vi "Subvi AO.vi"(2 "AO channel":refnum<k21>="Connector1/AO0", 10 "Memory label":refnum<k21>="AO0 buffer") -> ()   [LabVIEW 2017]
uses:
  <vilib>/rvi/Emulation/niFpgaGetClockAttributes.vi
  <vilib>/rvi/Emulation/niFpgaSctlEmulationGetInTimedLoop.vi
  <vilib>/rvi/Emulation/niFpgaEmulationReportErrorSimple.vi
  <vilib>/rvi/DataTransferAndStorage/Container/Common/niFpgaContainerExecOnDevCompGetState.vi
  <vilib>/rvi/Emulation/niFpgaEmulationIsFPGAContextNoSignature.vi
  <vilib>/rvi/DataTransferAndStorage/Container/Common/niFpgaContainerGetUniqueNameForEmu.vi
  <vilib>/rvi/Emulation/niFpgaProcessEmulError.vi
  <vilib>/rvi/errors/nirviReportUnexpectedCaseInternalError (U32).vi
  <vilib>/rvi/Memory/Memory_Emulation/niFpgaMemoryEmulationCacheClearOnFirstRun.vi
  <vilib>/rvi/Memory/Memory_Emulation/nirvimemoryEmulationManagerCache_MakeExclusive.vi
  <vilib>/rvi/Memory/Memory_Emulation/niFpgaMemoryEmulationValidateCache.vi
  <vilib>/rvi/Memory/Memory_Emulation/nirvimemoryEmulationManagerCache_InsertValue.vi
  <vilib>/Utility/error.llb/Clear Errors.vi
  <vilib>/rvi/Memory/Memory_Emulation/nirvimemoryEmulationManagerCache_ReleaseExclusive.vi
  <vilib>/rvi/Memory/Memory_Emulation/nirvimemoryEmulationManagerCache_GetValue.vi
  <vilib>/rvi/Memory/Memory_Emulation/nirvimemoryEmulationManagerCache_SetValue.vi
  <vilib>/rvi/Emulation/niFpgaSctlEmulationResourceMgr.vi
  <vilib>/rvi/eio/common/nirviEmuTemplateMethod_errors.vi
  GV trigger.vi
  <vilib>/rvi/Emulation/niFpgaCriticalErrorInLSC.vi
  <vilib>/rvi/DataTransferAndStorage/Container/XNode/niFpgaContainer.xnode
  <vilib>/rvi/Memory/Memory_Emulation/niFpgaMemoryEmulationRefIn.vi
  <vilib>/eio/EIONode/EIONode.xnode
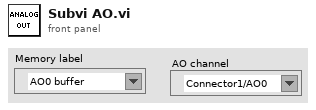
[diagram p1: front panel]
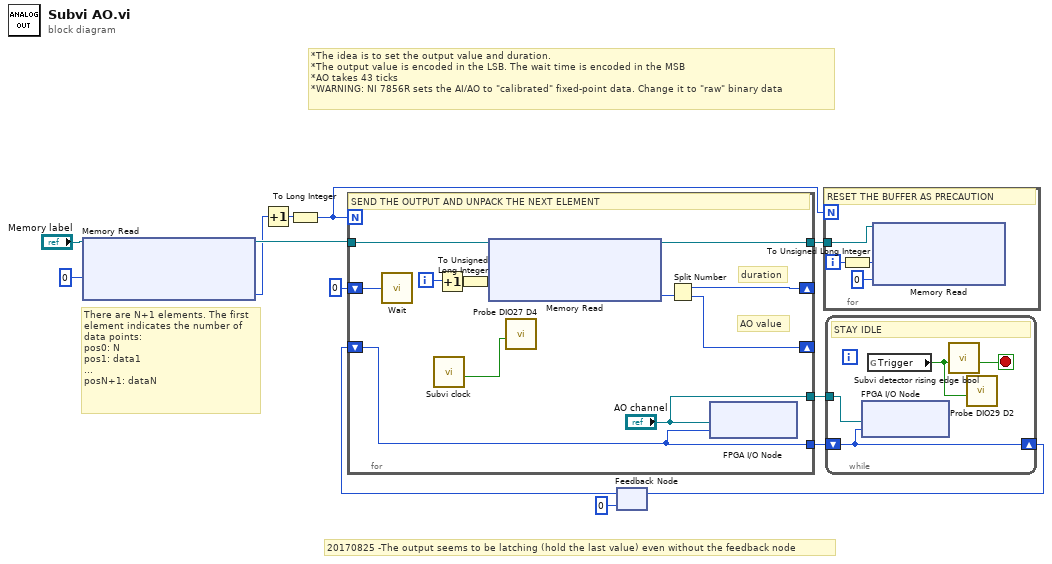
[diagram p0: block diagram]
diagram:
  # "20170825 -The output seems to be latching (hold the last value) even without the feedback node"
  # "There are N+1 elements. The first\nelement indicates the number of\ndata points:\npos0: N\npos1: data1\n...\nposN+1: dataN"
  # "*The idea is to set the output value and duration.\n*The output value is encoded in the LSB. The wait time is encoded in the MSB\n*AO takes 43 ticks\n*WARNING: NI 7856R sets the AI/AO to \"calibrated\" fixed-point data. Change it to \"raw\" binary data"
  n1 = xnode ("Memory Read")("Address"=u32 0, "Memory In"="Memory label") -> ("Data"=w7:u32, "Memory Out"=w9:refnum<k21>)
  n2 = Increment(x=w7) -> (x+1=w6:u32)
  n3 = To Long Integer(number=w6) -> (32bit integer=w5:i32)
  n4 = feedback #1(u16 0) -> (w3:u16)
  n5 = for {
    N: w5 -> [_]
    shift-right: [w24] -> _
    shift-left: u16 0 -> [w25]
    shift-right: [w22] -> _
    shift-left: w3 -> [w14]
    tunnel: ["AO channel"] -> w12
    tunnel: [w21] -> w8
    tunnel: w9 -> [w19]
    tunnel: [w14] -> w1
    i -> [w18]
    # "duration"
    # "AO value"
    # "SEND THE OUTPUT AND UNPACK THE NEXT ELEMENT"
    n6 = call "Wait"("Count(Ticks)"=w25) -> ()  [unwired: 1 out]
    n7 = call "Subvi clock.vi"() -> ("Output"=w15:bool)  [unwired: 11 in]
    n8 = Increment(x=w18) -> (x+1=w17:i32)
    n9 = To Unsigned Long Integer(number=w17) -> (unsigned 32bit integer=w16:u32)
    n10 = xnode ("Memory Read")("Memory In"=w19, "Address"=w16) -> ("Memory Out"=w21:refnum<k21>, "Data"=w23:u32)
    n11 = call "Probe DIO27 D4.vi"("D4"=w15) -> ()  [unwired: 11 in]
    n12 = Split Number(x=w23) -> (hi(x)=w24:u16, lo(x)=w22:u16)
    n13 = xnode "FPGA I/O Node"("I/O Item"=w14, "FPGA I/O In"="AO channel") -> ()  [unwired: 1 out]
  }
  n14 = for {
    N: w5 -> [_]
    tunnel: w8 -> [w29]
    i -> [w27]
    # "RESET THE BUFFER AS PRECAUTION"
    n15 = To Unsigned Long Integer(number=w27) -> (unsigned 32bit integer=w26:u32)
    n16 = xnode ("Memory Read")("Address"=w26, "Data"=u32 0, "Memory In"=w29) -> ()  [unwired: 1 out]
  }
  n17 = while {
    tunnel: w12 -> [w32]
    shift-right: [w31] -> w4
    shift-left: w1 -> [w31]
    stop <- w33 stop-if-true
    # "STAY IDLE"
    n18 = xnode "FPGA I/O Node"("I/O Item"=w31, "FPGA I/O In"=w32) -> ()  [unwired: 1 out]
    n19 = global read "GV trigger.vi" "Trigger"() -> (w30:bool)
    n20 = call "Subvi detector rising edge bool.vi"("Input"=w30) -> ("Output"=w33:bool)  [unwired: 10 in]
    n21 = call "Probe DIO29 D2.vi"("D2"=w30) -> ()  [unwired: 11 in]
  }
  n22 = feedback-in #1(w4) -> ()
